vi "Analysis.Convert Yields to Table.vi"(11 "Yields":T1) -> (3 "Table":string[][](table), 5 "Col Header":string[](array[string]))   [LabVIEW 2024]
uses:
  Analysis.Yield Info.ctl
  Analysis.Yield Info, Item.ctl
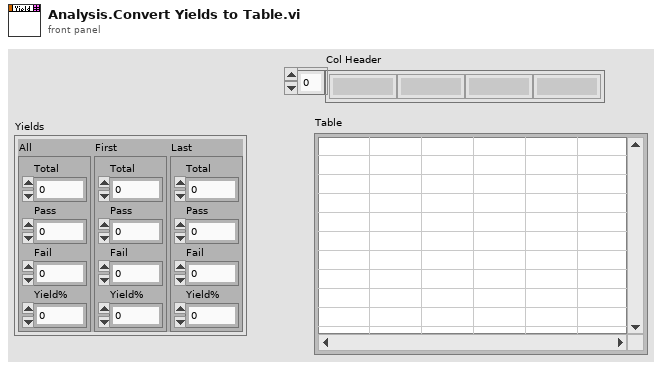
[diagram p1: front panel]
types:
  T1 = typedef "Analysis.Yield Info.ctl" = cluster{"All":T2, "First":T2, "Last":T2}
  T2 = typedef "Analysis.Yield Info, Item.ctl" = cluster{"Total":i32, "Pass":i32, "Fail":i32, "Yield%":dbl}
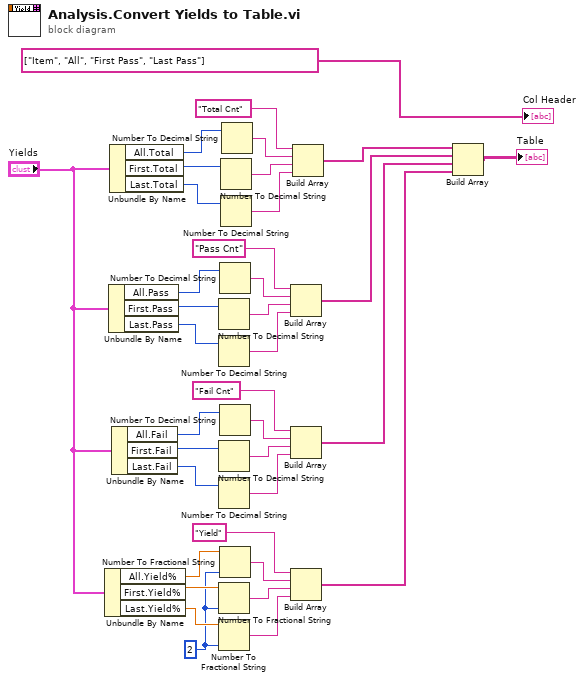
[diagram p0: block diagram]
diagram:
  w7 = i16 2 ("precision (6)")
  n1 = Unbundle By Name("Yields") -> ("All.Yield%"=w9:dbl, "First.Yield%"=w10:dbl, "Last.Yield%"=w11:dbl)
  n2 = Unbundle By Name("Yields") -> ("All.Pass"=w23:i32, "First.Pass"=w24:i32, "Last.Pass"=w25:i32)
  n3 = Unbundle By Name("Yields") -> ("All.Total"=w36:i32, "First.Total"=w35:i32, "Last.Total"=w34:i32)
  n4 = Unbundle By Name("Yields") -> ("All.Fail"=w22:i32, "First.Fail"=w21:i32, "Last.Fail"=w20:i32)
  n5 = Number To Decimal String(number=w24) -> (decimal integer string=w28:string)  [unwired: 1 in]
  n6 = Number To Decimal String(number=w25) -> (decimal integer string=w29:string)  [unwired: 1 in]
  n7 = Number To Decimal String(number=w21) -> (decimal integer string=w17:string)  [unwired: 1 in]
  n8 = Number To Decimal String(number=w20) -> (decimal integer string=w16:string)  [unwired: 1 in]
  n9 = Number To Fractional String(number=w10, precision (6)=w7) -> (F-format string=w14:string)  [unwired: 2 in]
  n10 = Number To Fractional String(number=w11, precision (6)=w7) -> (F-format string=w15:string)  [unwired: 2 in]
  n11 = Number To Decimal String(number=w23) -> (decimal integer string=w27:string)  [unwired: 1 in]
  n12 = Number To Decimal String(number=w22) -> (decimal integer string=w18:string)  [unwired: 1 in]
  n13 = Number To Fractional String(number=w9, precision (6)=w7) -> (F-format string=w13:string)  [unwired: 2 in]
  n14 = Number To Decimal String(number=w35) -> (decimal integer string=w31:string)  [unwired: 1 in]
  n15 = Number To Decimal String(number=w34) -> (decimal integer string=w30:string)  [unwired: 1 in]
  n16 = Number To Decimal String(number=w36) -> (decimal integer string=w32:string)  [unwired: 1 in]
  n17 = Build Array("Pass Cnt", w27, w28, w29) -> (w5:string[])
  n18 = Build Array("Fail Cnt", w18, w17, w16) -> (w4:string[])
  n19 = Build Array("Yield", w13, w14, w15) -> (w2:string[])
  n20 = Build Array("Total Cnt", w32, w31, w30) -> (w6:string[])
  n21 = Build Array(w6, w5, w4, w2) -> (→"Table":string[][])
  "Col Header" <- string[] ["Item", "All", "First Pass", "Last Pass"]
